vi "Write Publish Request Data.vi"(6 "Publisher ID":string, 8 "Publication Time":timestamp, 9 "Value":variant, 10 "Datum Name":string, 11 "PublishRequest In":refnum<class "PublishRequest.lvclass">) -> (3 "PublishRequest Out":refnum<class "PublishRequest.lvclass">)   [LabVIEW 2017, in "IMediator.lvlib" / "PublishRequest.lvclass"]
uses:
  PublishRequest.lvclass
  PublishRequest.lvclass/PublishRequest.ctl
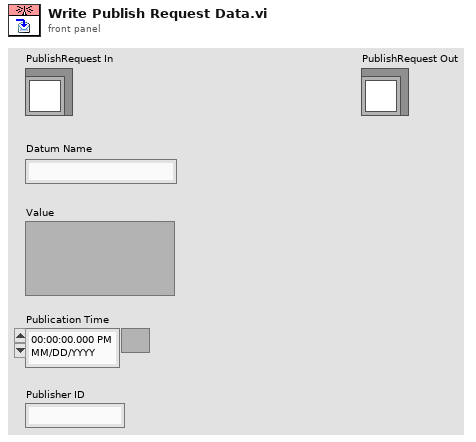
[diagram p1: front panel]
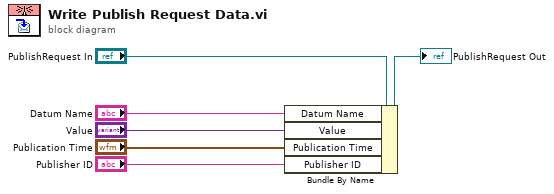
[diagram p0: block diagram]
diagram:
  n1 = Bundle By Name(cluster="PublishRequest In", "Datum Name"="Datum Name", "Value"="Value", "Publication Time"="Publication Time", "Publisher ID"="Publisher ID") -> (→"PublishRequest Out":refnum<class "PublishRequest.lvclass">)
